vi "Run Active Project Unit Tests.vi"(10 "Virtual Folder (empty: \"My Computer\")":string) -> ()   [LabVIEW 2013]
uses:
  classes/Test Runner.Project/Test Runner.Project.lvclass
  classes/Test Runner/Test Runner.lvclass
panel:
  out "error out":errorcluster
  # "CARAYA Run Active Project's Unit Tests\n\nThis tool will run all Caraya Unit Tests found in the active project."
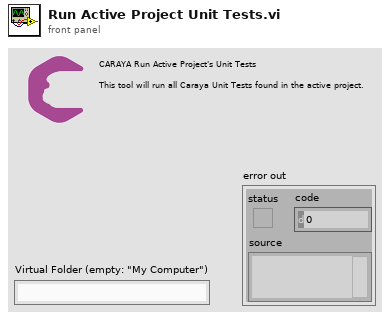
[diagram p1: front panel]
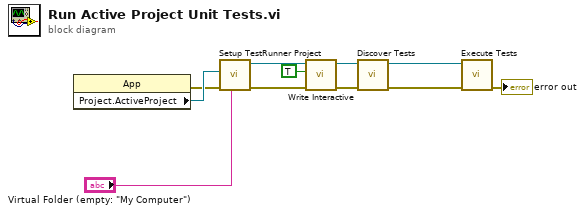
[diagram p0: block diagram]
diagram:
  n1 = property on="Property Node" class="App"() -> (error out=w7:errorcluster, "Project.ActiveProject"=w10:refnum<vi>)  [unwired: 2 in, 1 out]
  n2 = call "Setup TestRunner Project.vi"("Virtual Folder (empty: \"My Computer\")"="Virtual Folder (empty: \"My Computer\")", "error in (no error)"=w7, "Project Refnum"=w10) -> ("error out"=w9:errorcluster, "Test Runner.Project out"=w5:refnum<class "Test Runner.Project.lvclass">)  [unwired: 7 in]
  n3 = call "Write Interactive.vi"("Interactive"=TRUE, "Test Runner in"=w5) -> ("Test Runner out"=w4:refnum<class "Test Runner.Project.lvclass">)  [unwired: 9 in]
  n4 = call "Discover Tests.vi"("error in (no error)"=w9, "Test Runner in"=w4) -> ("error out"=w8:errorcluster, "Test Runner out"=w3:refnum<class "Test Runner.Project.lvclass">)  [unwired: 8 in]
  n5 = call-dynamic "Execute Tests.vi"("error in (no error)"=w8, "Test Runner in"=w3) -> ("error out"=→"error out":errorcluster)  [unwired: 8 in, 1 out]
